vi "Unforce Variable.vi"(0 "variable path (URL)":string, 11 "error in (no error)":errorcluster) -> (15 "error out":errorcluster)   [LabVIEW 2017]
doc: "Discontinues forcing on an I/O variable or I/O alias and returns control of the I/O value to the NI Scan Engine."
uses:
  <resource>/objmgr/ni.var.rc
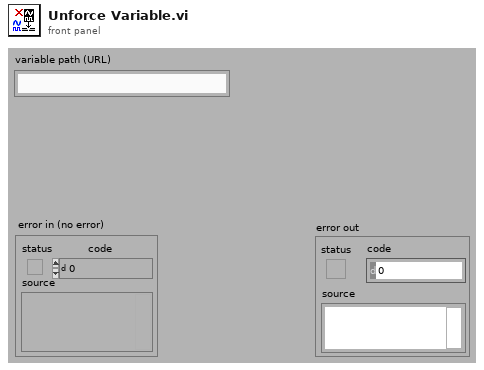
[diagram p1: front panel]
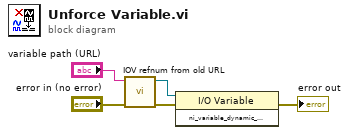
[diagram p0: block diagram]
diagram:
  n1 = call <vilib>:"IOV refnum from old URL.vi"("error in (no error)"="error in (no error)", "variable path (URL)"="variable path (URL)") -> ("error out"=w3:errorcluster, "IOV refnum"=w4:refnum<k21>)  [unwired: 8 in]
  n2 = invoke class="I/O Variable" method="ni_variable_dynamic_IOVariable_Unforce"(reference=w4, error in=w3) -> (error out=→"error out":errorcluster)  [unwired: 1 in, 2 out]
